vi "Extract waveform from numpy.ndarray.vi"(5 "I16":i16[](array[numeric])) -> (4 "Interleaved array":dbl[](array[numeric]), 6 "Complex array":cdb[](array[numeric]), 10 "2D-IQ":dbl[][](array[numeric]))   [LabVIEW 2019, in "mmW_commands.lvlib"]
uses:
  mmW_commands.lvlib
  commands/typedefs/datatypes_.ctl
panel:
  in  "error in":errorcluster
  out "error out":errorcluster
  in  "datatype":T1
  in  "flattened data":string
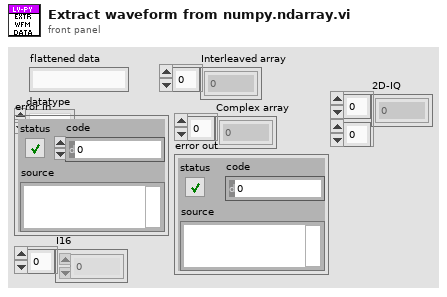
[diagram p1: front panel]
types:
  T1 = typedef "mmW_commands.lvlib/datatypes_.ctl" = enum16{"none", "string", "interleaved_I16", "interleaved_I32", "I16_array", "I32_array"}
  T2 = enum16{"big-endian, network order", "native, host order", "little-endian"}
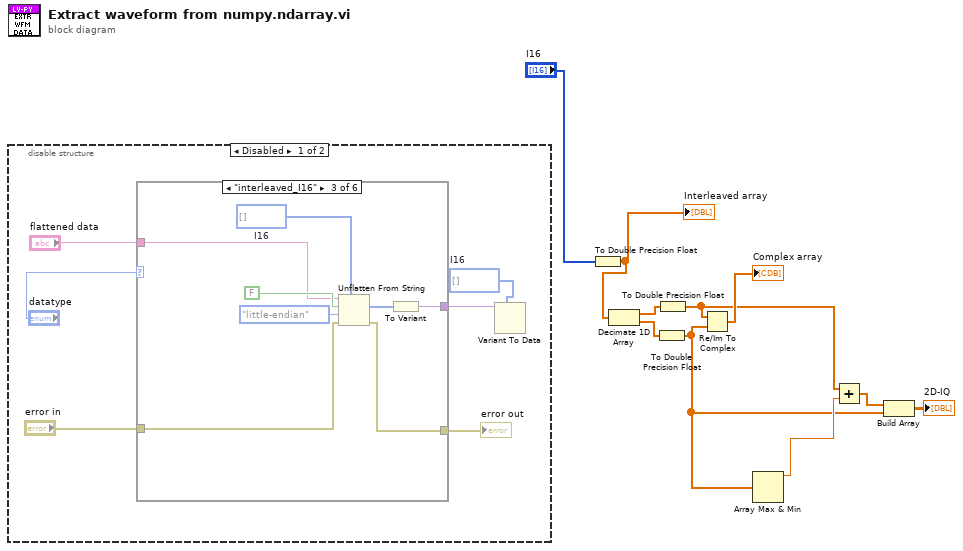
[diagram p0: block diagram]
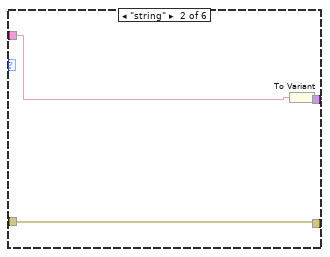
[diagram p3: hidden frame]
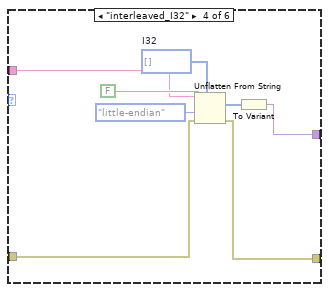
[diagram p4: hidden frame]
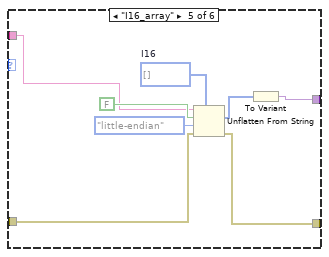
[diagram p5: hidden frame]
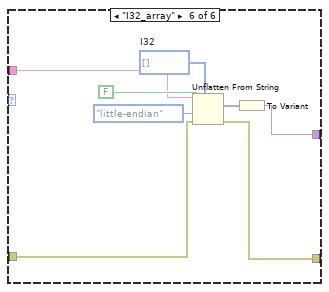
[diagram p6: hidden frame]
diagram:
  n1 = disable-structure shown="Disabled" {
    frame Disabled {
      w11 = i16[] []  # I16
      n2 = case shown="\"interleaved_I16\"" "datatype" {
        tunnel: "flattened data" -> [_ w20 w25 w32 w41 w48]
        tunnel: [_ w19 w23 w29 w39 w47] -> w15
        tunnel: "error in" -> [w17 w18 w22 w31 w38 w46]
        tunnel: [w17 w18 w21 w30 w37 w45] -> w12
        frame "none", Default {
        }
        frame "string" {
          n3 = To Variant(anything=w20) -> (Variant=w19:variant)
        }
        frame "interleaved_I16" {
          w28 = i16[] []  # I16
          n4 = Unflatten From String(type=w28, binary string=w25, data includes array or string size? (T)=FALSE, byte order (0:big-endian, network order)=T2."little-endian", error in (no error)=w22) -> (value=w24:i16[], error out=w21:errorcluster)  [unwired: 1 out]
          n5 = To Variant(anything=w24) -> (Variant=w23:variant)
        }
        frame "interleaved_I32" {
          w36 = i32[] []  # I32
          n6 = Unflatten From String(type=w36, binary string=w32, data includes array or string size? (T)=FALSE, byte order (0:big-endian, network order)=T2."little-endian", error in (no error)=w31) -> (value=w33:i32[], error out=w30:errorcluster)  [unwired: 1 out]
          n7 = To Variant(anything=w33) -> (Variant=w29:variant)
        }
        frame "I16_array" {
          w44 = i16[] []  # I16
          n8 = Unflatten From String(type=w44, binary string=w41, data includes array or string size? (T)=FALSE, byte order (0:big-endian, network order)=T2."little-endian", error in (no error)=w38) -> (value=w40:i16[], error out=w37:errorcluster)  [unwired: 1 out]
          n9 = To Variant(anything=w40) -> (Variant=w39:variant)
        }
        frame "I32_array" {
          w52 = i32[] []  # I32
          n10 = Unflatten From String(type=w52, binary string=w48, data includes array or string size? (T)=FALSE, byte order (0:big-endian, network order)=T2."little-endian", error in (no error)=w46) -> (value=w49:i32[], error out=w45:errorcluster)  [unwired: 1 out]
          n11 = To Variant(anything=w49) -> (Variant=w47:variant)
        }
      }
      "error out" <- w12
      n12 = Variant To Data(type=w11, Variant=w15) -> ()  [unwired: 1 in, 2 out]
    }
    frame Enabled {
    }
  }
  n13 = To Double Precision Float(number="I16") -> (double precision float=w7:dbl[])
  "Interleaved array" <- w7
  n14 = Decimate 1D Array(w7) -> (w10:dbl[], w9:dbl[])
  n15 = To Double Precision Float(number=w9) -> (double precision float=w2:dbl[])
  n16 = To Double Precision Float(number=w10) -> (double precision float=w4:dbl[])
  n17 = Re/Im To Complex(1:w2, 2:w4) -> (0:→"Complex array":cdb[])
  n18 = Array Max & Min(array=w2) -> (max value=w3:dbl)  [unwired: 3 out]
  n19 = Add(x=w4, y=w3) -> (x+y=w5:dbl[])
  n20 = Build Array(w5, w2) -> (→"2D-IQ":dbl[][])
